vi "Close Device.vi"(8 "error in (no error)":errorcluster, 11 "Handle":u64) -> (0 "error out":errorcluster)   [LabVIEW 2019, in "D2XX-lv.lvlib"]
doc: "Close an open device."
uses:
  D2XX-lv.lvlib
  <instrlib>/_D2XX/D2XX/D2XX.lvlib
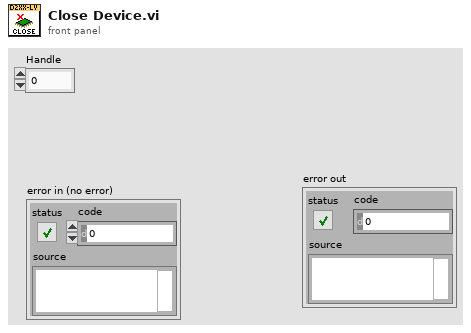
[diagram p1: front panel]
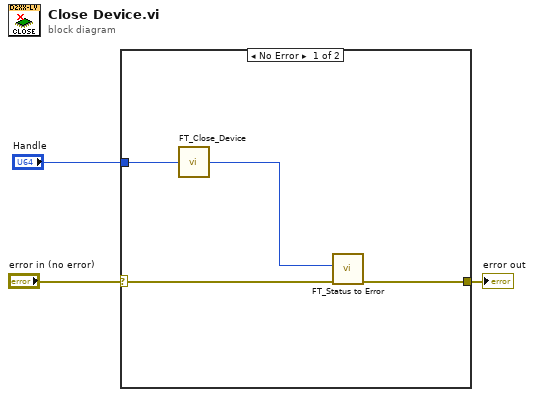
[diagram p0: block diagram]
diagram:
  n1 = case shown="No Error" "error in (no error)" {
    selector: "error in (no error)" -> [w7 w8]
    tunnel: [w6 w8] -> w2
    tunnel: "Handle" -> [w5 _]
    frame No Error {
      n2 = call <instrlib>:"FT_Close_Device.vi"("Handle"=w5) -> ("FT_Status"=w4:u32)
      n3 = call "FT_Status to Error.vi"("error in (no error)"=w7, "FT_Status"=w4) -> ("error out"=w6:errorcluster)  [unwired: 9 in]
    }
    frame Error {
    }
  }
  "error out" <- w2
